vi "Lobatto Quadrature Core (VI).vi"(7 "data":variant, 8 "tolerance":dbl=1e-10, 9 "lower limit":dbl, 10 "upper limit":dbl, 11 "f(x)":refnum<vi>) -> (0 "error out":errorcluster, 3 "result":dbl)   [LabVIEW 2017, in "NI_AALPro.lvlib"]
uses:
  <vilib>/Analysis/NI_AALPro.lvlib
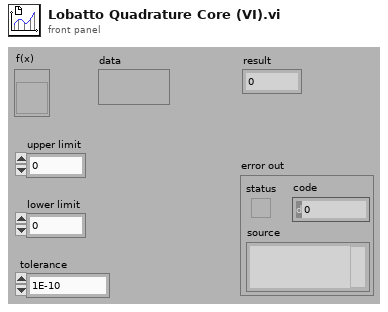
[diagram p1: front panel]
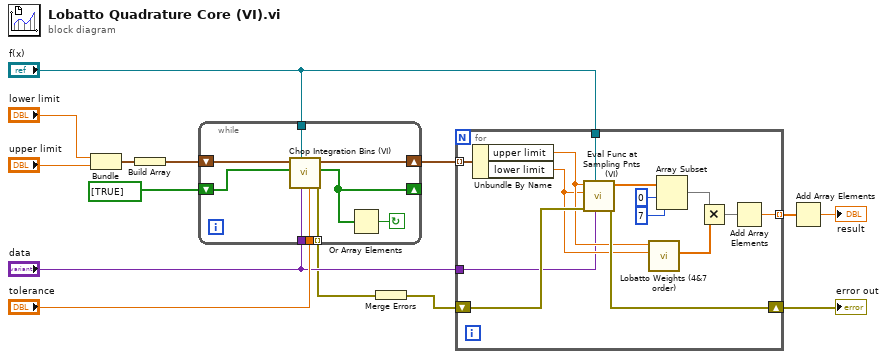
[diagram p0: block diagram]
diagram:
  n1 = Bundle("lower limit"="lower limit", "upper limit"="upper limit") -> (w12:cluster{"lower limit":dbl, "upper limit":dbl})  [unwired: 1 in]
  n2 = Build Array(w12) -> (w11:cluster{"lower limit":dbl, "upper limit":dbl}[])
  n3 = while {
    shift-right: [w20] -> w10
    shift-left: w11 -> [w22]
    shift-right: [w19] -> _
    shift-left: bool[] [TRUE] ("appended array") -> [w21]
    tunnel: [w18] -> w2 mode=indexing
    tunnel: "tolerance" -> [w17]
    tunnel: "f(x)" -> [w16]
    tunnel: "data" -> [w15]
    stop <- w23 continue-if-true
    n4 = call <vilib>:"Chop Integration Bins (VI).vi"("tolerance"=w17, "data"=w15, "f(x)"=w16, "Chop In"=w21, "Bins In"=w22) -> ("error out"=w18:errorcluster, "Chop Out"=w19:bool[], "Bins Out"=w20:cluster{"lower limit":dbl, "upper limit":dbl}[])  [unwired: 4 in]
    n5 = Or Array Elements(Boolean array=w19) -> (logical OR=w23:bool)
  }
  n6 = Merge Errors(w2) -> (w1:errorcluster)
  n7 = for {
    tunnel: w10 -> [w36] mode=indexing
    tunnel: [w37] -> w9 mode=indexing
    shift-right: [w30] -> w5
    shift-left: w1 -> [w29]
    tunnel: "f(x)" -> [w25]
    tunnel: "data" -> [w24]
    n8 = Unbundle By Name(w36) -> ("upper limit"=w28:dbl, "lower limit"=w27:dbl)
    n9 = call <vilib>:"Eval Func at Sampling Pnts (VI).vi"("data"=w24, "f(x)"=w25, "error in (no error)"=w29, "lower limit"=w27, "upper limit"=w28) -> ("error out"=w30:errorcluster, "Function Evaluations (7 and 4 pts)"=w26:dbl[])  [unwired: 4 in, 1 out]
    n10 = call <vilib>:"Lobatto Weights (4&7 order).vi"("lower limit"=w27, "upper limit"=w28) -> ("Weights (7-Order)"=w35:dbl[])  [unwired: 8 in, 1 out]
    n11 = Array Subset(array=w26, index=0, length=7) -> (w34:dbl[])
    n12 = Multiply(x=w34, y=w35) -> (x*y=w31:dbl[])
    n13 = Add Array Elements(numeric array=w31) -> (sum=w37:dbl)
  }
  "error out" <- w5
  n14 = Add Array Elements(numeric array=w9) -> (sum=→"result":dbl)
